vi "ProtoTracking_Velocity.vi"() -> ()   [LabVIEW 2015]
uses:
  <vilib>/userdefined/High Color/IMAQdx.ctl
  <vilib>/vision/driver/NI_Vision_Acquisition_Software.lvlib
  <vilib>/vision/NI_Vision_Development_Module.lvlib
  <userlib>/Newport ESP301/Newport ESP301.lvlib
panel:
  in  "Move":bool
  out "Image":T1(plugin-control)
  out "Centroid":cluster{"X Centroid":sgl, "Y Centroid":sgl} {"Y Centroid" format="%.2f"; "X Centroid" format="%.2f"}
  in  "Stop Button":bool
  in  "Camera Name":T2="cam0"
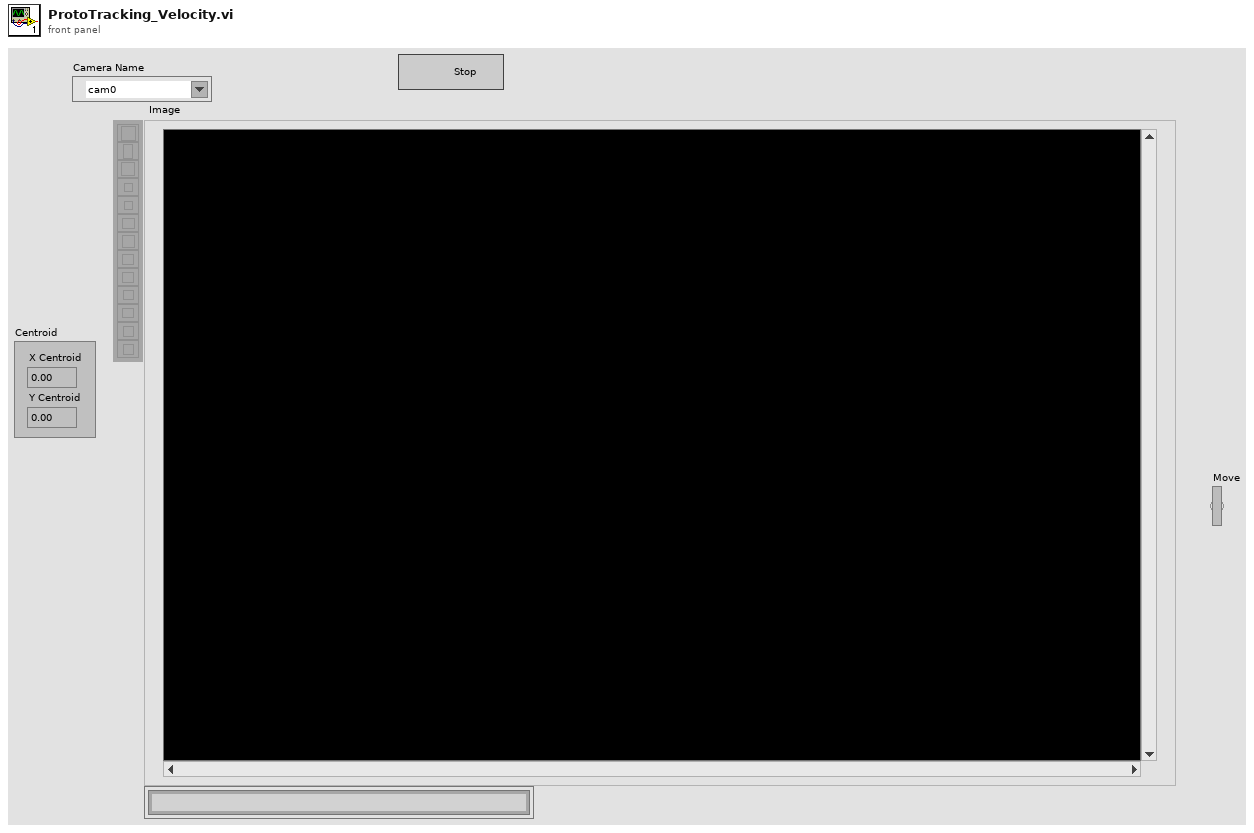
[diagram p1: front panel]
types:
  T1 = typedef "IMAQ Image.ctl" = refnum<image>
  T2 = typedef "IMAQdx.ctl" = refnum<k21>
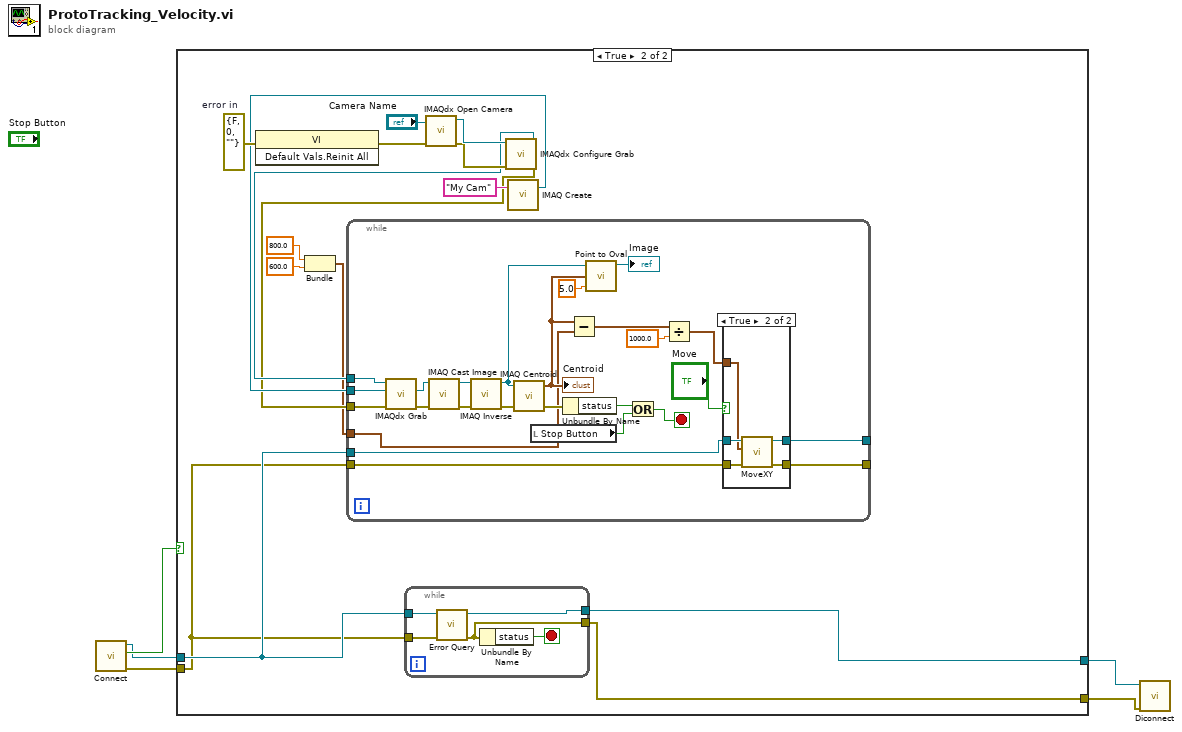
[diagram p0: block diagram]
diagram:
  n1 = call "Connect.vi"() -> ("error out"=w3:errorcluster, "Connected"=w5:bool, "VISA resource name out"=w4:refnum<visa-resource-name>)  [unwired: 5 in]
  n2 = case shown="True" w5 {
    tunnel: w4 -> [w6 w11]
    tunnel: w3 -> [w7 w10]
    tunnel: [w6 w9] -> w2
    tunnel: [w7 w8] -> w1
    frame False {
    }
    frame True {
      w22 = errorcluster {"status"=FALSE, "code"=0, "source"=""}  # error in
      n3 = invoke class="VI" method="Default Vals.Reinit All"(error in=w22) -> (error out=w21:errorcluster)  [unwired: 2 in, 2 out]
      n4 = Bundle(800.0, 600.0) -> (w12:cluster{dbl, dbl})  [unwired: 1 in]
      n5 = while {
        tunnel: w11 -> [w28]
        tunnel: w10 -> [w27]
        tunnel: [w25] -> w9
        tunnel: [w24] -> w8
        stop <- w26 stop-if-true
        n6 = call <userlib>:"Error Query.vi"("error in (no error)"=w27, "VISA resource name"=w28) -> ("error out"=w24:errorcluster, "VISA resource name out"=w25:refnum<visa-resource-name>)  [unwired: 2 in, 2 out]
        n7 = Unbundle By Name(w24) -> ("status"=w26:bool)
      }
      n8 = call <vilib>:"IMAQdx Open Camera.vi"("error in"=w21, "Session In"="Camera Name") -> ("error out"=w18:errorcluster, "Session Out"=w19:T2)  [unwired: 8 in]
      n9 = call <vilib>:"IMAQdx Configure Grab.vi"("error in"=w18, "Session In"=w19) -> ("error out"=w15:errorcluster, "Session Out"=w17:T2)  [unwired: 8 in]
      n10 = call "IMAQ Create"("Image Name"="My Cam") -> ("New Image"=w16:T1)  [unwired: 4 in, 1 out]
      n11 = while {
        tunnel: w17 -> [w53]
        tunnel: w16 -> [w52]
        tunnel: w15 -> [w51]
        tunnel: w11 -> [w32]
        tunnel: w10 -> [w31]
        tunnel: [w34] -> _
        tunnel: [w33] -> _
        tunnel: w12 -> [w37]
        stop <- w48 stop-if-true
        n12 = call <vilib>:"IMAQdx Grab.vi"("error in"=w51, "Image In"=w52, "Session In"=w53) -> ("error out"=w45:errorcluster, "Image Out"=w46:T1)  [unwired: 5 in, 2 out]
        n13 = call "IMAQ Cast Image"("error in (no error)"=w45, "Image Src"=w46) -> ("error out"=w42:errorcluster, "Image Dst Out"=w40:T1)  [unwired: 8 in]
        n14 = call "IMAQ Inverse"("error in (no error)"=w42, "Image Src"=w40) -> ("error out"=w41:errorcluster, "Image Dst Out"=w39:T1)  [unwired: 8 in]
        n15 = call "IMAQ Centroid"("error in (no error)"=w41, "Image"=w39) -> ("error out"=w47:errorcluster, "Centroid"=w38:cluster{"X Centroid":sgl, "Y Centroid":sgl})  [unwired: 2 in]
        "Centroid" <- w38
        n16 = local read "Stop Button"() -> (w49:bool)
        n17 = Unbundle By Name(w47) -> ("status"=w50:bool)
        n18 = Subtract(x=w38, y=w37) -> (x-y=w36:cluster{dbl, dbl})
        n19 = call "Point to Oval.vi"("Image In"=w39, "Point"=w38, "Size"=5.0) -> ("Image Out"=→"Image":T1)  [unwired: 3 in]
        n20 = Or(x=w50, y=w49) -> (x .or. y?=w48:bool)
        n21 = Divide(x=w36, y=1000.0) -> (x/y=w30:cluster{dbl, dbl})
        n22 = case shown="True" "Move" {
          tunnel: [w55 w60] -> w34
          tunnel: [w54 w59] -> w33
          tunnel: w32 -> [w55 w58]
          tunnel: w31 -> [w54 w57]
          tunnel: w30 -> [_ w56]
          frame False {
          }
          frame True {
            n23 = call "MoveXY.vi"("error in (no error)"=w57, "XY Cluster"=w56, "VISA resource name"=w58) -> ("error out"=w59:errorcluster, "VISA resource Out"=w60:refnum<visa-resource-name>)  [unwired: 7 in]
          }
        }
      }
    }
  }
  n24 = call "Diconnect.vi"("error in (no error)"=w1, "VISA resource name"=w2) -> ()  [unwired: 6 in]
